vi "SaccadeAnalyser - Make Traces Positive.vi"(8 "error in (no error)":errorcluster, 9 "enum_direction":enum16{"Positive", "Negative"}(ring) caption="Impulse Direction", 10 "Response in":dbl[](array[numeric]), 11 "Stimulus in":dbl[](array[numeric])) -> (0 "error out":errorcluster, 2 "Response out":dbl[](array[numeric]), 3 "Stimulus out":dbl[](array[numeric]))   [LabVIEW 2016]
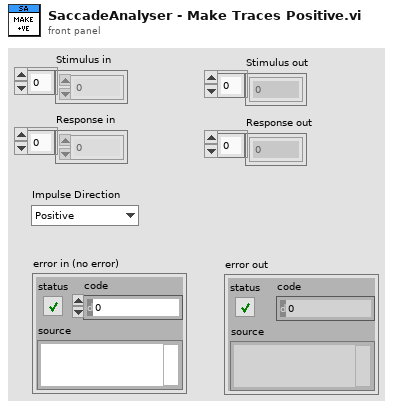
[diagram p1: front panel]
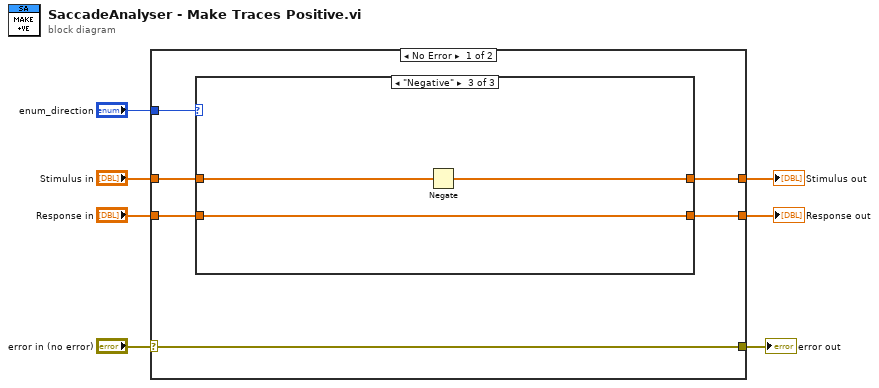
[diagram p0: block diagram]
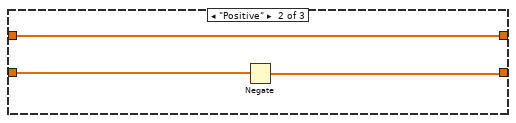
[diagram p3: hidden frame]
diagram:
  n1 = case shown="No Error" "error in (no error)" {
    selector: "error in (no error)" -> [w8 w22]
    tunnel: "Stimulus in" -> [w12 w24]
    tunnel: "Response in" -> [w11 w23]
    tunnel: "enum_direction" -> [w13 _]
    tunnel: [w10 w24] -> w2
    tunnel: [w9 w23] -> w1
    tunnel: [w8 w22] -> w3
    frame No Error {
      n2 = case shown="\"Negative\"" w13 {
        tunnel: w12 -> [w15 w18 w20]
        tunnel: w11 -> [w14 w17 w21]
        tunnel: [w15 w18 w19] -> w10
        tunnel: [w14 w16 w21] -> w9
        frame Default {
        }
        frame "Positive" {
          n3 = Negate(x=w17) -> (-x=w16:dbl[])
        }
        frame "Negative" {
          n4 = Negate(x=w20) -> (-x=w19:dbl[])
        }
      }
    }
    frame Error {
    }
  }
  "Stimulus out" <- w2
  "Response out" <- w1
  "error out" <- w3
